vi "Fix CLFN Paths.vi"(8 "error in (no error)":errorcluster, 11 "Library Ref":refnum<vi>) -> (0 "error out":errorcluster, 3 "Library Ref Out":refnum<vi>)   [LabVIEW 2020]
doc: "Fixes up the path in all Call Library Function Nodes within the library. This needs to be done after a copy of the library has been saved, else all CLFN will still point to the original library.\n\nAssumes shared libraries are in the library, and not simply included as a dependency."
uses:
  <vilib>/Utility/traverseref.llb/TRef TravTarget.ctl
  <vilib>/Utility/traverseref.llb/VI Scripting - Traverse.lvlib
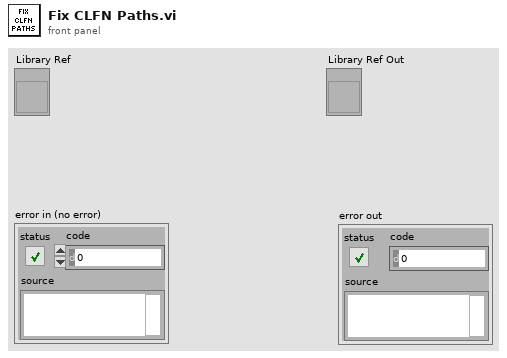
[diagram p1: front panel]
types:
  T1 = typedef "TRef TravTarget.ctl" = enum16{"FP", "BD", "Other"}
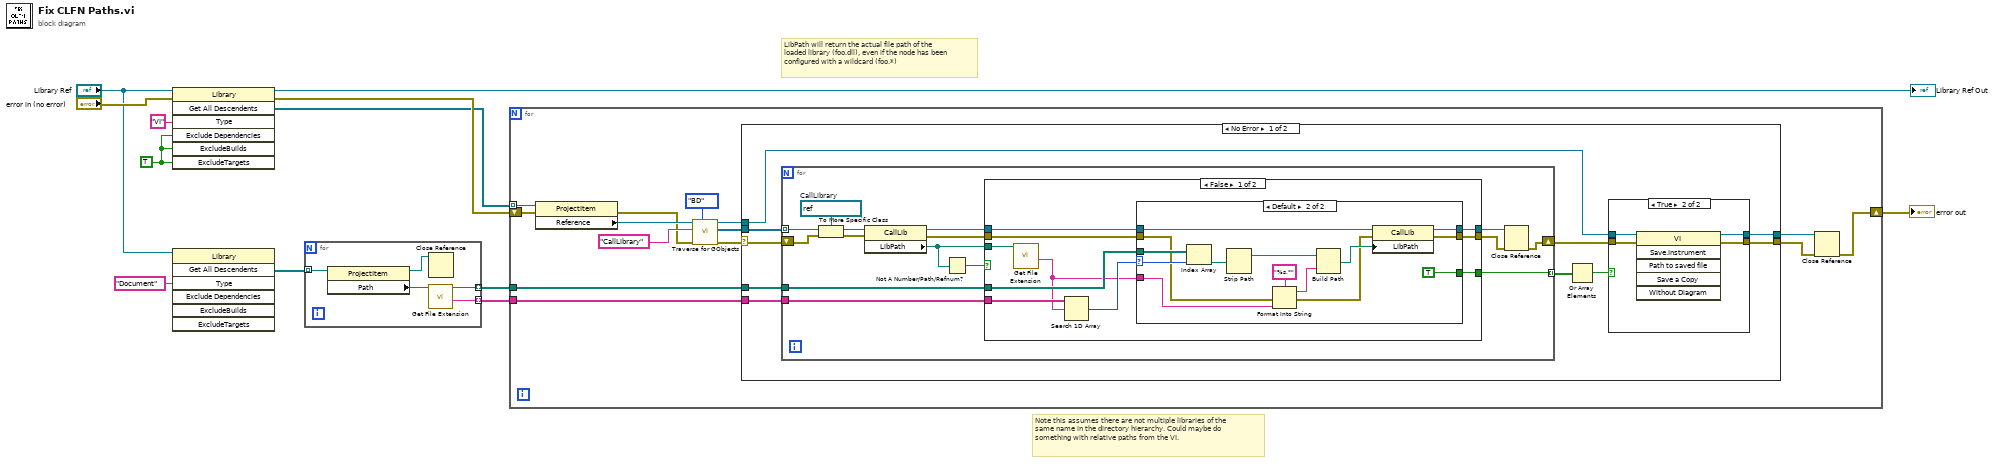
[diagram p0: block diagram]
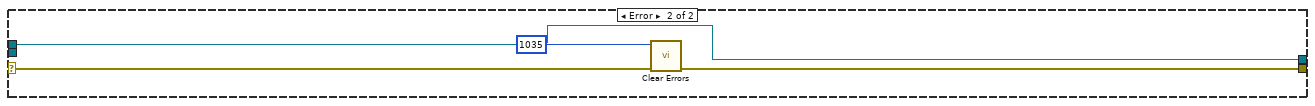
[diagram p5: hidden frame]
diagram:
  w12 = TRUE ("ExcludeDependencies")
  # "Note this assumes there are not multiple libraries of the same name in the directory hierarchy. Could maybe do something with relative paths from the VI."
  # "LibPath will return the actual file path of the loaded library (foo.dll), even if the node has been configured with a wildcard (foo.*)"
  n1 = invoke class="Library" method="Get All Descendents"(reference="Library Ref", error in="error in (no error)", "Type"="VI", "Exclude Dependencies"=w12, "ExcludeBuilds"=w12, "ExcludeTargets"=w12) -> (reference out=→"Library Ref Out":refnum<vi>, error out=w9:errorcluster, "All Descendents"=w8:refnum<vi>[])  [unwired: 1 in, 4 out]
  n2 = invoke class="Library" method="Get All Descendents"(reference="Library Ref", "Type"="Document") -> ("All Descendents"=w4:refnum<vi>[])  [unwired: 5 in, 6 out]
  n3 = for {
    tunnel: w4 -> [w17] mode=indexing
    tunnel: [w14] -> w2 mode=indexing
    tunnel: [w16] -> w1 mode=indexing
    n4 = property class="ProjectItem"(reference=w17) -> (reference out=w13:refnum<vi>, "Path"=w15:path)  [unwired: 1 in, 1 out]
    n5 = call <vilib>:"Get File Extension.vi"("file"=w15) -> ("filename without extension"=w16:string, "dup file"=w14:path)  [unwired: 6 in, 3 out]
    n6 = Close Reference(reference=w13) -> ()  [unwired: 1 in, 1 out]
  }
  n7 = for {
    tunnel: w8 -> [w31] mode=indexing
    shift-right: [w22] -> w3
    shift-left: w9 -> [w27]
    tunnel: w2 -> [w26]
    tunnel: w1 -> [w20]
    n8 = property class="ProjectItem"(reference=w31, error in=w27) -> (error out=w18:errorcluster, "Reference"=w19:refnum<vi>)  [unwired: 1 out]
    n9 = call <vilib>:"Traverse for GObjects.vi"("Traverse Target"=TRef_TravTarget."BD", "error in (no error)"=w18, "Class Name"="CallLibrary", "VI Refnum"=w19) -> ("error out"=w21:errorcluster, "References"=w28:refnum<vi>[], "dup VI Refnum"=w25:refnum<vi>)  [unwired: 4 in, 1 out]
    n10 = case shown="No Error" w21 {
      selector: w21 -> [w33 w94]
      tunnel: w28 -> [w41 _]
      tunnel: w26 -> [w40 _]
      tunnel: w25 -> [w39 w91]
      tunnel: [w37 w91] -> w24
      tunnel: [w36 w92] -> w23
      tunnel: w20 -> [w32 _]
      frame No Error {
        n11 = for {
          tunnel: w41 -> [w56] mode=indexing
          shift-right: [w44] -> w38
          shift-left: w33 -> [w53]
          tunnel: w40 -> [w47]
          tunnel: [w43] -> w35 mode=indexing
          tunnel: w32 -> [w42]
          w55 = refnum<vi> refnum  # CallLibrary
          n12 = To More Specific Class(target class=w55, reference=w56, error in=w53) -> (specific class reference=w54:refnum<vi>, error out=w52:errorcluster)
          n13 = property class="CallLib"(reference=w54, error in=w52) -> (reference out=w49:refnum<vi>, error out=w50:errorcluster, "LibPath"=w48:path)
          n14 = Not A Number/Path/Refnum?(number/path/refnum=w48) -> (NaN/Path/Refnum?=w51:bool)
          n15 = case shown="False" w51 {
            tunnel: w50 -> [w59 w83]
            tunnel: w49 -> [w66 w84]
            tunnel: w48 -> [w58 _]
            tunnel: w47 -> [w60 _]
            tunnel: [w65 w83] -> w45
            tunnel: [w64 w84] -> w46
            tunnel: [w63 _] -> w43
            tunnel: w42 -> [w62 _]
            frame False {
              n16 = call <vilib>:"Get File Extension.vi"("file"=w58) -> ("filename without extension"=w57:string)  [unwired: 6 in, 4 out]
              n17 = Search 1D Array(1D array=w62, element=w57) -> (index of element=w61:i32)  [unwired: 1 in]
              n18 = case shown="Default" w61 {
                selector: w61 -> [_ w71]
                tunnel: w66 -> [w68 w82]
                tunnel: w59 -> [w67 w70]
                tunnel: w60 -> [_ w81]
                tunnel: [w67 w74] -> w65
                tunnel: [w68 w73] -> w64
                tunnel: [_ TRUE] -> w63
                tunnel: w57 -> [_ w69]
                frame -1 {
                }
                frame Default {
                  n19 = Index Array(array=w81, index=w71) -> (element=w80:path)
                  n20 = Strip Path(path=w80) -> (stripped path=w78:path)  [unwired: 1 out]
                  n21 = Format Into String(format string="%s.*", error in=w70, w69) -> (resulting string=w77:string, error out=w75:errorcluster)  [unwired: 1 in]
                  n22 = Build Path(base path=w78, name or relative path=w77) -> (appended path=w76:path)
                  n23 = property class="CallLib"(reference=w82, error in=w75, "LibPath"=w76) -> (reference out=w73:refnum<vi>, error out=w74:errorcluster)
                }
              }
            }
            frame True {
            }
          }
          n24 = Close Reference(reference=w46, error in (no error)=w45) -> (error out=w44:errorcluster)
        }
        n25 = Or Array Elements(Boolean array=w35) -> (logical OR=w34:bool)
        n26 = case shown="True" w34 {
          tunnel: w39 -> [w86 w90]
          tunnel: w38 -> [w85 w89]
          tunnel: [w86 w88] -> w37
          tunnel: [w85 w87] -> w36
          frame False {
          }
          frame True {
            n27 = invoke class="VI" method="Save.Instrument"(reference=w90, error in=w89) -> (reference out=w88:refnum<vi>, error out=w87:errorcluster)  [unwired: 4 in, 4 out]
          }
        }
      }
      frame Error {
        n28 = call <vilib>:"Clear Errors.vi"("error in (no error)"=w94, "specific error code to clear (0: all)"=1035) -> ("error out"=w92:errorcluster)  [unwired: 4 in, 1 out]
      }
    }
    n29 = Close Reference(reference=w24, error in (no error)=w23) -> (error out=w22:errorcluster)
  }
  "error out" <- w3
